vi "scan.step.vi"(6 "ScanWhat?":enum16{"Nothing", "Lumonics", "Delay"}(ring), 8 "inhibit\nstep":bool, 9 "Mono":T2={"offset (cm-1)"=200.0, "step (cm-1)"=2.0, "Counter"=146.4557703573521, "Scanstep/monostep"=20, "Status"={"Moving"=FALSE, "Home"=FALSE, "Hi"=FALSE, "Low"=FALSE}, "nm"=585.8230814294084, "Mono port"="COM7"}, 10 "DyeLaser":T4={"Scan.Start (cm-1)"=15000.0, "Scan.Stop (cm-1)"=15050.0, "Scan.step (cm-1)"=0.2, "dye laser port"="", "Laser"=enum."Syrah", "NSteps"=251, "CurrentStep"=75, "Current.cm-1"=15015.0} {"Current.cm-1" format="%.2f"}, 11 "Camera":T3={"Gate.Delay"=0, "Delay.Step"=0, "Gate.Duration"=150000, "#Accum"=10, "SetpointTemp"=-30, "Last Temp"=6, "Current Temp"=4}) -> (1 "Mono.out":T1, 2 "DyeLaser out":T4={"Scan.Start (cm-1)"=15000.0, "Scan.Stop (cm-1)"=15050.0, "Scan.step (cm-1)"=0.2, "dye laser port"="", "Laser"=enum."Syrah", "NSteps"=251, "CurrentStep"=75, "Current.cm-1"=15015.0} {"Current.cm-1" format="%.2f"}, 3 "Camera out":T3)   [LabVIEW 2022 SP3]
panel:
  # "ns"
  # "ns"
  # "ns"
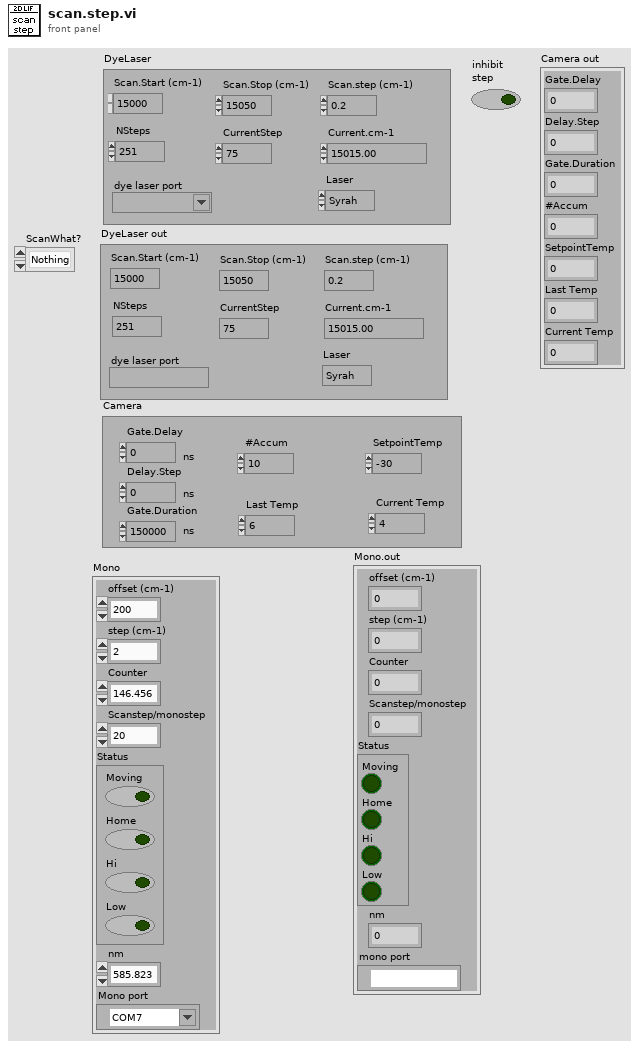
[diagram p1: front panel]
types:
  T1 = cluster{"offset (cm-1)":dbl, "step (cm-1)":dbl, "Counter":dbl, "Scanstep/monostep":i32, "Status":cluster{"Moving":bool, "Home":bool, "Hi":bool, "Low":bool}, "nm":dbl, "mono port":refnum<visa-resource-name>}
  T2 = cluster{"offset (cm-1)":dbl, "step (cm-1)":dbl, "Counter":dbl, "Scanstep/monostep":i32, "Status":cluster{"Moving":bool, "Home":bool, "Hi":bool, "Low":bool}, "nm":dbl, "Mono port":refnum<visa-resource-name>}
  T3 = cluster{"Gate.Delay":u64, "Delay.Step":u64, "Gate.Duration":u64, "#Accum":i32, "SetpointTemp":i32, "Last Temp":i32, "Current Temp":i32}
  T4 = cluster{"Scan.Start (cm-1)":dbl, "Scan.Stop (cm-1)":dbl, "Scan.step (cm-1)":dbl, "dye laser port":refnum<visa-resource-name>, "Laser":enum16{"Syrah", "Hyperdye"}, "NSteps":i32, "CurrentStep":i32, "Current.cm-1":dbl}
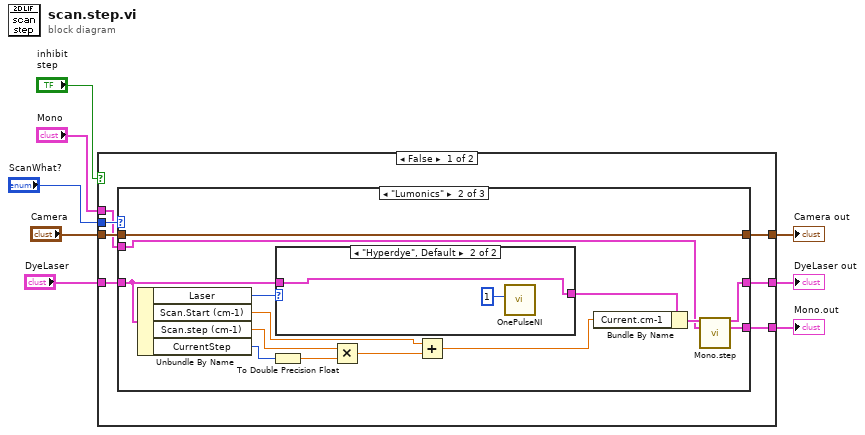
[diagram p0: block diagram]
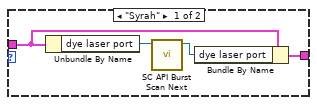
[diagram p3: hidden frame]
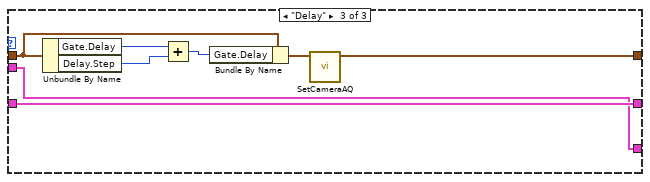
[diagram p4: hidden frame]
diagram:
  n1 = case shown="False" "inhibit\nstep" {
    tunnel: [w15 w49] -> w8
    tunnel: "DyeLaser" -> [w11 w49]
    tunnel: "Camera" -> [w12 w48]
    tunnel: [w14 w48] -> w4
    tunnel: "ScanWhat?" -> [w13 _]
    tunnel: "Mono" -> [w10 w47]
    tunnel: [w9 w47] -> w1
    frame False {
      n2 = case shown="\"Lumonics\"" w13 {
        tunnel: [w18 w20 w41] -> w15
        tunnel: w11 -> [w18 w24 w41]
        tunnel: w12 -> [w17 w23 w45]
        tunnel: [w17 w23 w42] -> w14
        tunnel: w10 -> [w16 w21 w39]
        tunnel: [w16 w19 w39] -> w9
        frame "Nothing", Default {
        }
        frame "Lumonics" {
          n3 = Unbundle By Name(w24) -> ("Laser"=w26:enum16{"Syrah", "Hyperdye"}, "Scan.Start (cm-1)"=w30:dbl, "Scan.step (cm-1)"=w27:dbl, "CurrentStep"=w28:i32)
          n4 = To Double Precision Float(number=w28) -> (double precision float=w32:dbl)
          n5 = case shown="\"Hyperdye\", Default" w26 {
            tunnel: w24 -> [w34 w37]
            tunnel: [w35 w37] -> w25
            frame "Syrah" {
              n6 = Unbundle By Name(w34) -> ("dye laser port"=w36:refnum<visa-resource-name>)
              n7 = call "SC API Burst Scan Next.vi"("VISA Resource Name"=w36) -> ("VISA Resource Name Out"=w33:refnum<visa-resource-name>)  [unwired: 9 in, 1 out]
              n8 = Bundle By Name(cluster=w34, "dye laser port"=w33) -> (w35:T4)
            }
            frame "Hyperdye", Default {
              n9 = call "OnePulseNI.vi"("pulse width ms"=u32 1) -> ()  [unwired: 11 in]
            }
          }
          n10 = Multiply(x=w27, y=w32) -> (x*y=w29:dbl)
          n11 = Add(x=w30, y=w29) -> (x+y=w31:dbl)
          n12 = Bundle By Name(cluster=w25, "Current.cm-1"=w31) -> (w22:T4)
          n13 = call "Mono.step.vi"("DyeLaser"=w22, "Mono"=w21) -> ("DyeLaser out"=w20:T4, "Mono.out"=w19:T1)  [unwired: 12 in]
        }
        frame "Delay" {
          n14 = Unbundle By Name(w45) -> ("Gate.Delay"=w46:u64, "Delay.Step"=w40:u64)
          n15 = Add(x=w46, y=w40) -> (x+y=w44:u64)
          n16 = Bundle By Name(cluster=w45, "Gate.Delay"=w44) -> (w43:T3)
          n17 = call "SetCameraAQ.vi"("Camera"=w43) -> ("Camera out"=w42:T3)  [unwired: 9 in, 1 out]
        }
      }
    }
    frame True {
    }
  }
  "DyeLaser out" <- w8
  "Camera out" <- w4
  "Mono.out" <- w1
